vi "TestMan-Simple Chat.vi"() -> ()   [LabVIEW 2016]
panel:
  out "Array (log)":string[](array[string])
  in  "Transmit":bool
  in  "message":string[](array[string])
  out "ID not the same!":bool
  out "ServerID out":u8
  out "status":bool
  in  "Stopp":bool
  in  "id in":u8=1
  in  "type in":u8=150
  in  "ttl in":u32=1
  in  "port in":u32=50000
  in  "ipadress in":string="224.5.6.7"
  # "UDP-network"
  # "TestMan Settings"
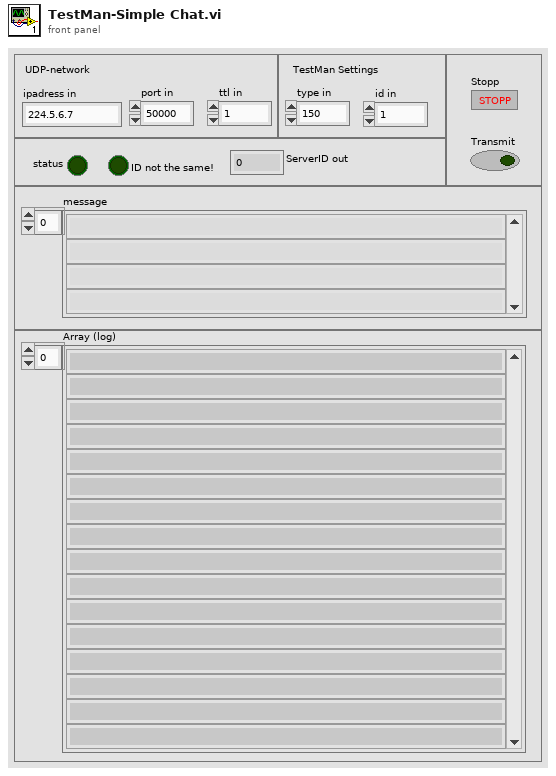
[diagram p1: front panel]
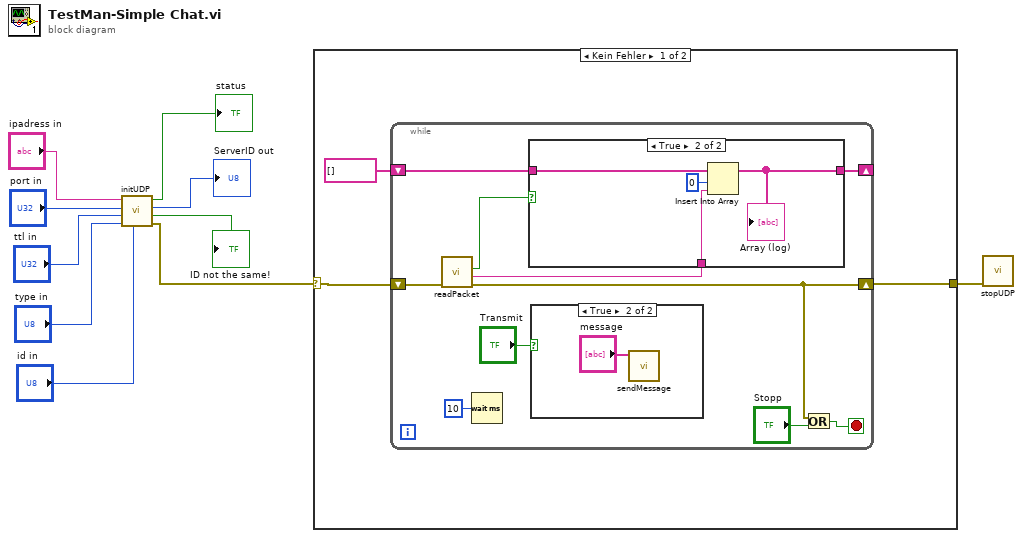
[diagram p0: block diagram]
diagram:
  n1 = call "initUDP.vi"("id in"="id in", "type in"="type in", "ttl in"="ttl in", "port in"="port in", "ipadress in"="ipadress in") -> ("error out"=w5:errorcluster, "ID not the same!"=→"ID not the same!":bool, "ServerID out"=→"ServerID out":u8, "status"=→"status":bool)  [unwired: 2 in]
  n2 = case shown="Kein Fehler" w5 {
    selector: w5 -> [w13 w30]
    tunnel: [w11 w30] -> w1
    frame No Error {
      n3 = while {
        shift-right: [w18] -> w11
        shift-left: w13 -> [w21]
        shift-right: [w16] -> _
        shift-left: string[] [] ("Array") -> [w17]
        stop <- w20 stop-if-true
        n4 = call "readPacket.vi"("error in (no error)"=w21) -> ("error out"=w18:errorcluster, "string"=w15:string, "data_available"=w14:bool)  [unwired: 5 in, 1 out]
        n5 = Wait (ms)(milliseconds to wait=u32 10 ("Zu wartende ms")) -> ()  [unwired: 1 out]
        n6 = case shown="True" w14 {
          tunnel: w17 -> [w24 w28]
          tunnel: [w24 w27] -> w16
          tunnel: w15 -> [_ w26]
          frame False {
          }
          frame True {
            n7 = Insert Into Array(array=w28, index=0 ("Index"), new element=w26) -> (w27:string[])
            "Array (log)" <- w27
          }
        }
        n8 = case shown="True" "Transmit" {
          frame False {
          }
          frame True {
            n9 = call "sendMessage.vi"("message"="message") -> ()  [unwired: 9 in, 2 out]
          }
        }
        n10 = Or(x=w18, y="Stopp") -> (x .or. y?=w20:bool)
      }
    }
    frame Error {
    }
  }
  n11 = call "stopUDP.vi"("error in (no error)"=w1) -> ()  [unwired: 10 in, 1 out]
